vi "Write Binary Reply Messages.vi"(9 "Error Msg":refnum<class "Message.lvclass">, 10 "No Error Msg":refnum<class "Message.lvclass">, 11 "BinaryDecisionMsg in":refnum<class "BinaryDecisionMsg.lvclass">) -> (3 "BinaryDecisionMsg out":refnum<class "BinaryDecisionMsg.lvclass">)   [LabVIEW 2015, in "AbstractMessages.lvlib" / "BinaryDecisionMsg.lvclass"]
uses:
  BinaryDecisionMsg.lvclass
  <vilib>/ActorFramework/Message/Message.lvclass
  BinaryDecisionMsg.lvclass/BinaryDecisionMsg.ctl
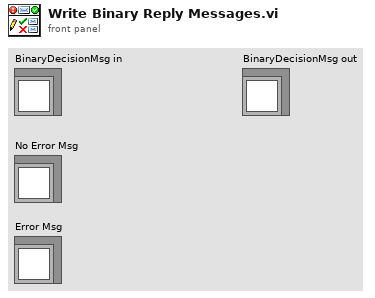
[diagram p1: front panel]
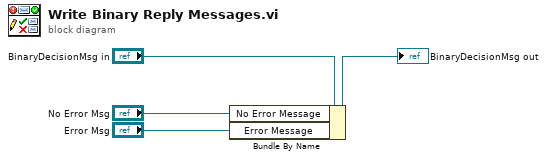
[diagram p0: block diagram]
diagram:
  n1 = Bundle By Name(cluster="BinaryDecisionMsg in", "No Error Message"="No Error Msg", "Error Message"="Error Msg") -> (→"BinaryDecisionMsg out":refnum<class "BinaryDecisionMsg.lvclass">)
